vi "Initialize.vi"(8 "error in":errorcluster, 11 "Report Generator in":refnum<class "Report Generator.lvclass">) -> (0 "error out":errorcluster, 3 "Report Generator out":refnum<class "Report Generator.lvclass">)   [LabVIEW 2023, in "Report Generator.lvlib" / "Report Generator.lvclass"]
uses:
  Library/Report Generator.lvclass
  C:/Users/Public/Documents/Development/builds/Engine/Engine.lvlibp/Project/Engine.lvclass
  builds/Tools/Config.lvlibp/Config.lvclass
  Library/Report Generator.lvclass/Report Generator.ctl
  Accessors/Read Report.vi
  builds/Engine/Engine.lvlibp/Accessors/Read Directory.vi
  builds/Tools/Report.lvlibp/Report.lvclass
  builds/Engine/Engine.lvlibp/Project/Engine.lvclass
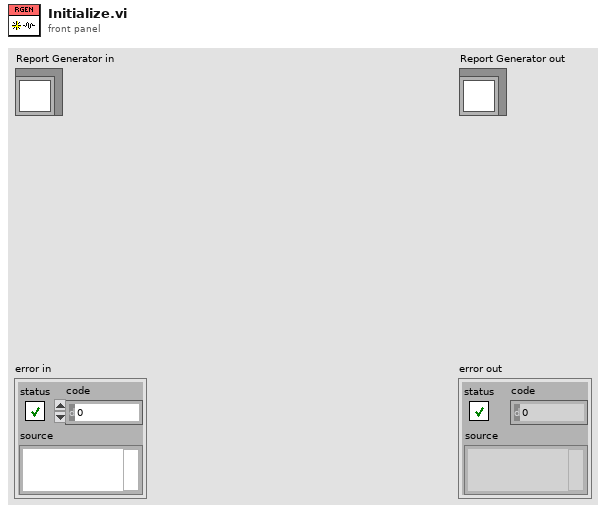
[diagram p1: front panel]
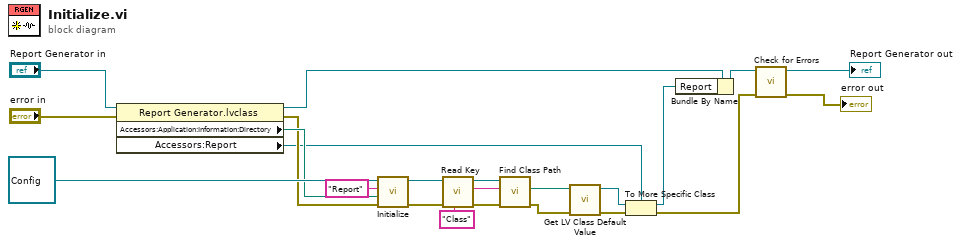
[diagram p0: block diagram]
diagram:
  n1 = property class="Report Generator.lvclass"(reference="Report Generator in", error in="error in") -> (reference out=w19:refnum<class "Report Generator.lvclass">, error out=w7:errorcluster, "Accessors:Application:Information:Directory"=w15:path, "Accessors:Report"=w3:refnum<class "Report.lvclass">)
  n2 = call-dynamic "Initialize.vi"("error in"=w7, "Path"=w15, "Device"="Report", "Config in"=refnum<class "Config.lvclass"> refnum) -> ("error out"=w14:errorcluster, "Config out"=w18:refnum<class "Config.lvclass">)  [unwired: 6 in]
  n3 = call "Read Key.vi"("Key Name"="Class", "error in"=w14, "Config in"=w18) -> ("error out"=w10:errorcluster, "Key Value"=w11:string, "Config out"=w12:refnum<class "Config.lvclass">)  [unwired: 6 in]
  n4 = call "Find Class Path.vi"("error in"=w10, "Class Name"=w11, "Config in"=w12) -> ("error out"=w8:errorcluster, "Class Path"=w9:path)  [unwired: 6 in, 1 out]
  n5 = call <vilib>:"Get LV Class Default Value.vi"("error in (no error)"=w8, "class path"=w9) -> ("error out"=w4:errorcluster, "object"=w5:refnum<class>)  [unwired: 8 in]
  n6 = To More Specific Class(target class=w3, reference=w5, error in=w4) -> (specific class reference=w2:refnum<class "Report.lvclass">, error out=w1:errorcluster)
  n7 = Bundle By Name(cluster=w19, "Report"=w2) -> (w6:refnum<class "Report Generator.lvclass">)
  n8 = call "Check for Errors.vi"("error in"=w1, "Engine in"=w6) -> ("error out"=→"error out":errorcluster, "Engine in"=→"Report Generator out":refnum<class "Report Generator.lvclass">)  [unwired: 8 in]
